vi "Get Type.vi"() -> (3 "Node Result":T1)   [LabVIEW 2013, in "Caraya.lvlib" / "Test Result.lvclass"]
uses:
  Test Result.lvclass
  Node Results.ctl
  Test Node.ctl
  Test Registration Data.ctl
  Assert Event Data.ctl
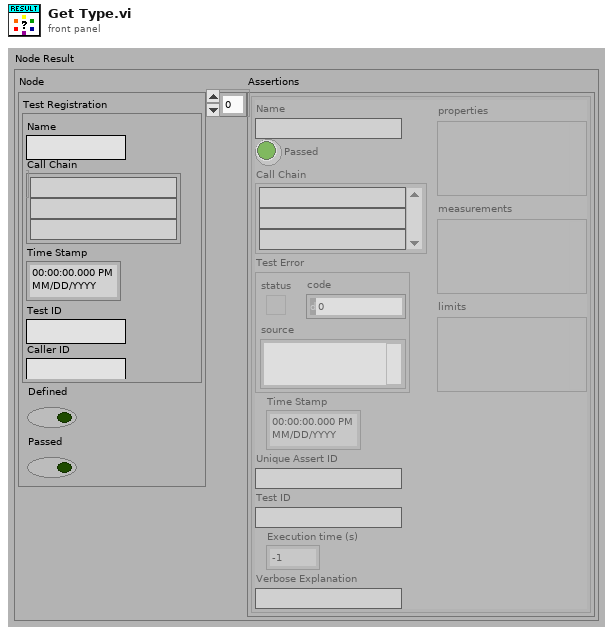
[diagram p1: front panel]
types:
  T1 = typedef "Caraya.lvlib/Test Result.lvclass/Node Results.ctl" = cluster{"Node":T2, "Assertions":T4[]}
  T2 = typedef "Caraya.lvlib/Test Result.lvclass/Test Node.ctl" = cluster{"Test Registration":T3, "Defined":bool, "Passed":bool}
  T3 = typedef "Caraya.lvlib/Test Result.lvclass/Test Registration Data.ctl" = cluster{"Name":string, "Call Chain":string[], "Time Stamp":timestamp, "Test ID":string, "Caller ID":string}
  T4 = typedef "Caraya.lvlib/Test Result.lvclass/Assert Event Data.ctl" = cluster{"Name":string, "Passed":bool, "Call Chain":string[], "Test Error":errorcluster, "Time Stamp":timestamp, "Unique Assert ID":string, "Test ID":string, "Execution time (s)":dbl, "Verbose Explanation":string, "properties":variant, "measurements":variant, "limits":variant}
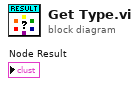
[diagram p0: block diagram]
diagram:
